vi "Destroy.vi"(0 "reference in":refnum<class "File Controller.lvclass">, 5 "error in (no error)":errorcluster) -> (14 "reference out":refnum<class "File Controller.lvclass">, 19 "error out":errorcluster)   [LabVIEW 2015, in "File Controller.lvclass"]
doc: "Destructor."
uses:
  File Controller.lvclass
  <vilib>/addons/_AddQ/G#Object/G#Object.lvclass
  APP/python_class/python.lvclass
  APP/excelFile_class/excelFile.lvclass
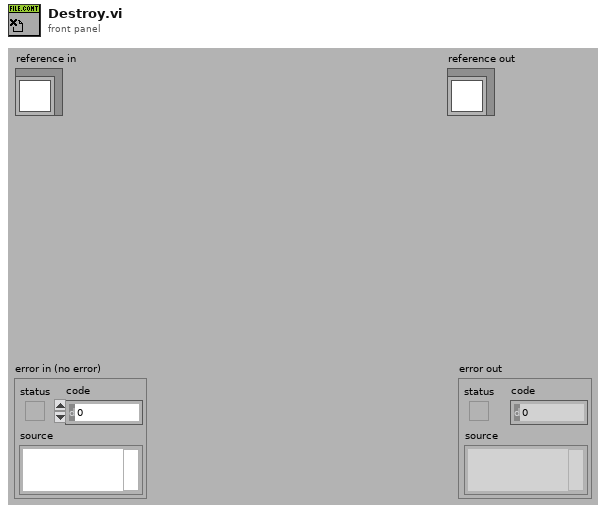
[diagram p1: front panel]
types:
  T1 = typedef "File Controller.lvclass/ObjectAttributes.ctl" = cluster{"MyAttribute":dbl, "excelFile_refs":refnum<class "excelFile.lvclass">[], "filePaths":path[], "outlookTemplatePaths":path[], "attachmentTemplatePaths":path[], "configFilePath":path, "not_setting":bool[], "python_ref":refnum<class "python.lvclass">}
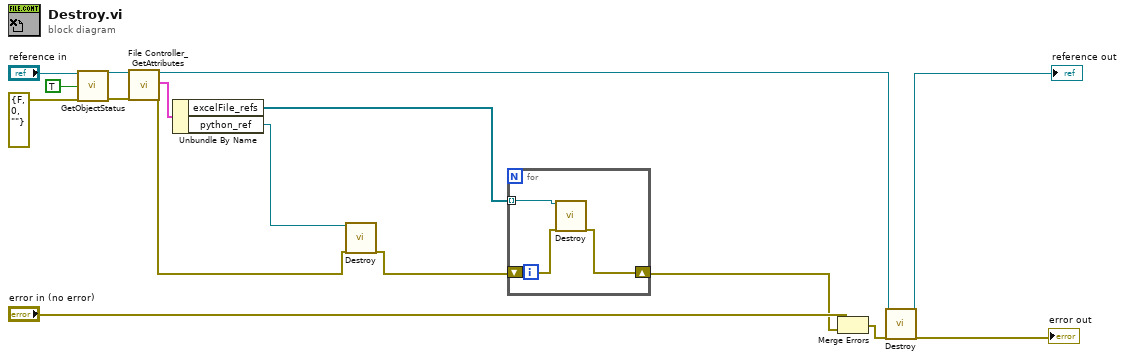
[diagram p0: block diagram]
diagram:
  n1 = call-dynamic "GetObjectStatus.vi"("reference in"="reference in", "simple info (F)"=TRUE ("simple info"), "error in (no error)"=errorcluster {"status"=FALSE, "code"=0, "source"=""}) -> ("reference out"=w10:refnum<class "File Controller.lvclass">, "error out"=w11:errorcluster)  [unwired: 5 in, 10 out]
  n2 = call "File Controller_GetAttributes.vi"("reference in"=w10, "error in (no error)"=w11) -> ("reference out"=w9:refnum<class "File Controller.lvclass">, "attributes"=w8:T1, "error out"=w2:errorcluster)  [unwired: 14 in, 1 out]
  n3 = Unbundle By Name(w8) -> ("excelFile_refs"=w5:refnum<class "excelFile.lvclass">[], "python_ref"=w3:refnum<class "python.lvclass">)
  n4 = call-dynamic "Destroy.vi"("reference in"=w3, "error in (no error)"=w2) -> ("error out"=w1:errorcluster)  [unwired: 16 in, 1 out]
  n5 = for {
    tunnel: w5 -> [w17] mode=indexing
    shift-right: [w18] -> w4
    shift-left: w1 -> [w19]
    n6 = call-dynamic "Destroy.vi"("reference in"=w17, "error in (no error)"=w19) -> ("error out"=w18:errorcluster)  [unwired: 16 in, 1 out]
  }
  n7 = Merge Errors("error in (no error)", w4) -> (w15:errorcluster)
  n8 = call-parent "Destroy.vi"("reference in"=w9, "error in (no error)"=w15) -> ("reference out"=→"reference out":refnum<class "File Controller.lvclass">, "error out"=→"error out":errorcluster)  [unwired: 16 in]
